vi "scan2d_initialize_log.vi"(8 "error in (no error)":errorcluster, 11 "scan_2d in":refnum<class "scan_2d.lvclass">) -> (0 "error out":errorcluster, 3 "scan_2d out":refnum<class "scan_2d.lvclass">)   [LabVIEW 2015, in "scan_2d.lvclass"]
uses:
  scan_2d.lvclass
  scan_2d.lvclass/scan_2d.ctl
  scan_2d_hdf5_log/scan_2d_hdf5_log.lvclass
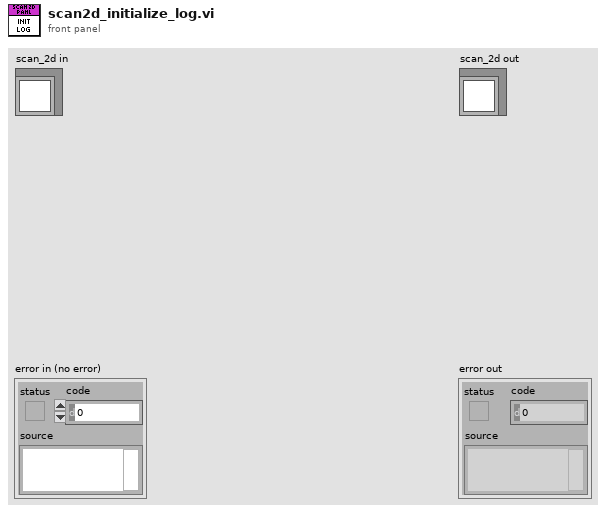
[diagram p1: front panel]
types:
  T1 = cluster{"x_positions":dbl[], "y_positions":dbl[]}
  T2 = typedef "data_types_tdef.ctl" = enum16{"0D", "1D", "2D"}
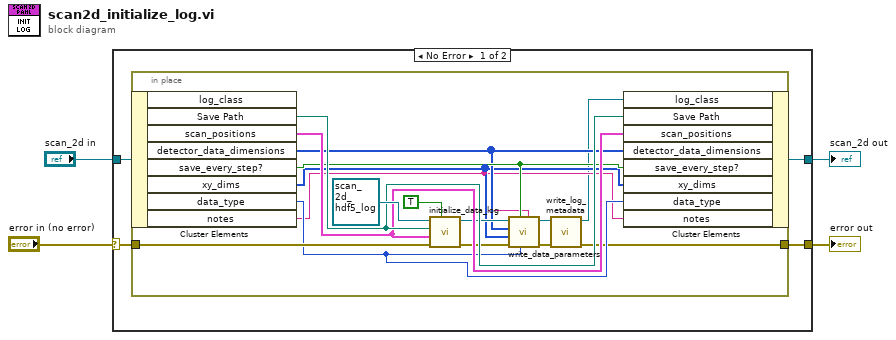
[diagram p0: block diagram]
diagram:
  n1 = case shown="No Error" "error in (no error)" {
    selector: "error in (no error)" -> [w7 w26]
    tunnel: [w6 w26] -> w3
    tunnel: [w5 w25] -> w1
    tunnel: "scan_2d in" -> [w8 w25]
    frame No Error {
      n2 = in-place {
        in-place-border: w7 -> [w23]
        in-place-border: [w9] -> w6
        n3 = in-place-cluster #1(w8) -> ("Save Path"=w22:path, "scan_positions"=w20:T1, "detector_data_dimensions"=w16:u32[], "save_every_step?"=w17:bool, "xy_dims"=w14:u32[], "data_type"=w15:T2, "notes"=w13:string)  [unwired: 1 out]
        n4 = call-dynamic "initialize_data_log.vi"("Overwrite?"=TRUE, "error in (no error)"=w23, "Initialization Data"=w20, "Path"=w22, "scan_hdf5_log in"=refnum<class "scan_2d_hdf5_log.lvclass"> refnum) -> ("error out"=w18:errorcluster, "scan_hdf5_log out"=w19:refnum<class "scan_2d_hdf5_log.lvclass">)  [unwired: 5 in]
        n5 = call "write_data_parameters.vi"("Notes"=w13, "data_type"=w15, "save_every_step?"=w17, "error in (no error)"=w18, "xy_dims"=w14, "detector_data_dimensions"=w16, "scan_2d_hdf5_log in"=w19) -> ("error out"=w12:errorcluster, "scan_2d_hdf5_log out"=w11:refnum<class "scan_2d_hdf5_log.lvclass">)  [unwired: 3 in]
        n6 = call-dynamic "write_log_metadata.vi"("error in (no error)"=w12, "scan_hdf5_log in"=w11) -> ("error out"=w9:errorcluster, "scan_hdf5_log out"=w10:refnum<class "scan_2d_hdf5_log.lvclass">)  [unwired: 8 in]
        n7 = in-place-cluster #1("log_class"=w10, "Save Path"=w22, "scan_positions"=w20, "detector_data_dimensions"=w16, "save_every_step?"=w17, "xy_dims"=w14, "data_type"=w15, "notes"=w13) -> (w5:refnum<class "scan_2d.lvclass">)
      }
    }
    frame Error {
    }
  }
  "error out" <- w3
  "scan_2d out" <- w1
